vi "for_v0_v12.vi"() -> ()   [LabVIEW 2009]
panel:
  out "Nr":dbl=1.0
  in  "Start":bool=TRUE
  in  "stop":bool
  out "Gauge":dbl(knob)=2.0 scale=0.0..9.0
  out "L6":bool
  out "L4":bool=TRUE
  out "L5":bool=TRUE
  out "L7":bool=TRUE
  out "L3":bool=TRUE
  out "L2":bool
  out "L1":bool=TRUE
  # "Stop"
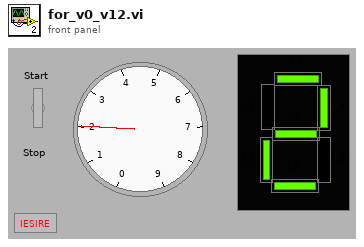
[diagram p1: front panel]
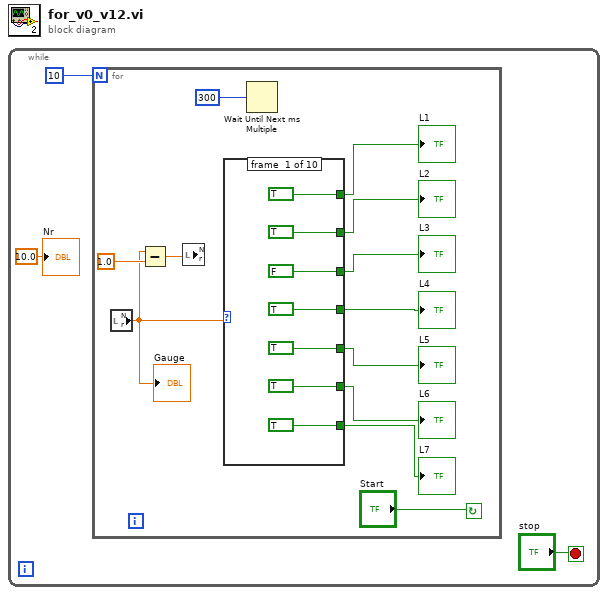
[diagram p0: block diagram]
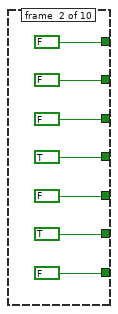
[diagram p2: hidden frame]
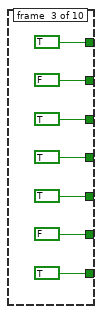
[diagram p3: hidden frame]
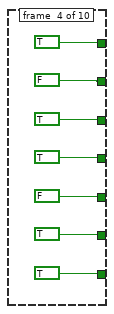
[diagram p4: hidden frame]
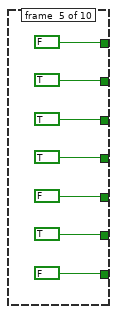
[diagram p5: hidden frame]
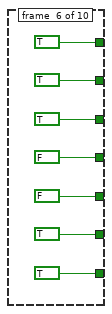
[diagram p6: hidden frame]
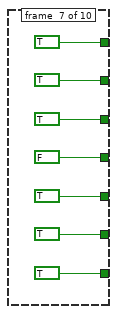
[diagram p7: hidden frame]
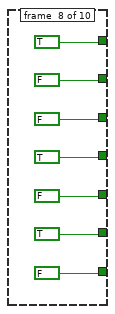
[diagram p8: hidden frame]
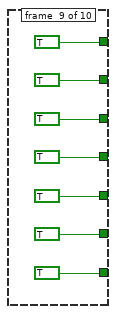
[diagram p9: hidden frame]
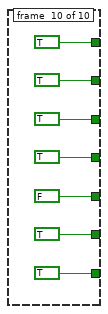
[diagram p10: hidden frame]
diagram:
  n1 = while {
    stop <- "stop" stop-if-true
    n2 = for {
      N: 10 -> [_]
      stop <- "Start" continue-if-true
      n3 = local read "Nr"() -> (w4:dbl)
      "Gauge" <- w4
      n4 = Subtract(x=w4, y=1.0 ("x")) -> (x-y=w6:dbl)
      n5 = local write "Nr"(w6) -> ()
      n6 = case shown="8" w4 {
        tunnel: [TRUE FALSE TRUE TRUE FALSE TRUE TRUE TRUE TRUE TRUE] -> w15
        tunnel: [TRUE FALSE FALSE FALSE TRUE TRUE TRUE FALSE TRUE TRUE] -> w14
        tunnel: [FALSE FALSE TRUE TRUE TRUE TRUE TRUE FALSE TRUE TRUE] -> w13
        tunnel: [TRUE TRUE TRUE TRUE TRUE FALSE FALSE TRUE TRUE TRUE] -> w12
        tunnel: [TRUE FALSE TRUE FALSE FALSE FALSE TRUE FALSE TRUE FALSE] -> w11
        tunnel: [TRUE TRUE FALSE TRUE TRUE TRUE TRUE TRUE TRUE TRUE] -> w10
        tunnel: [TRUE FALSE TRUE TRUE FALSE TRUE TRUE FALSE TRUE TRUE] -> w9
        frame #0 {
        }
        frame #1 {
        }
        frame #2 {
        }
        frame #3 {
        }
        frame #4 {
        }
        frame #5 {
        }
        frame #6 {
        }
        frame #7 {
        }
        frame #8 {
        }
        frame #9 {
        }
      }
      "L1" <- w15
      "L2" <- w14
      "L3" <- w13
      "L7" <- w9
      "L5" <- w11
      "L4" <- w12
      "L6" <- w10
      n7 = Wait Until Next ms Multiple(millisecond multiple=u32 300 ("milliseconds to wait")) -> ()  [unwired: 1 out]
    }
    "Nr" <- 10.0 ("Nr")
  }
